vi "Config data to StepData.vi"(11 "Data":string[](array[string])) -> (3 "RootStepData":string[](array[string]))   [LabVIEW 2021, in "DataBase_SQL.lvclass"]
uses:
  <userlib>/John_Lib/DataBase/DataBase_SQL/DataBase_SQL.lvclass
  <userlib>/John_Lib/DataBase/DataBase_SQL/DataBase_SQL.lvclass/DataBase_SQL.ctl
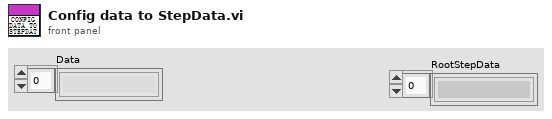
[diagram p1: front panel]
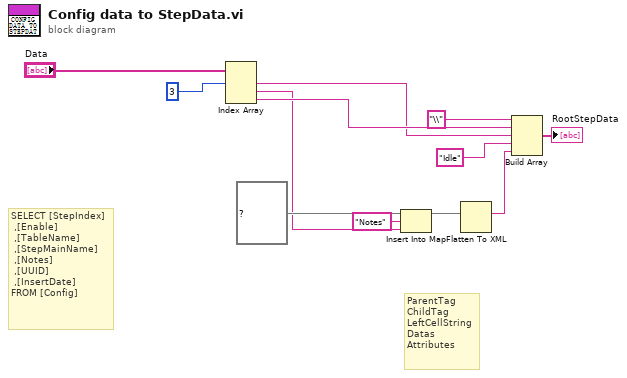
[diagram p0: block diagram]
diagram:
  # "SELECT [StepIndex]\n\t,[Enable]\n\t,[TableName]\n\t,[StepMainName]\n\t,[Notes]\n\t,[UUID]\n\t,[InsertDate]\nFROM [Config]"
  # "ParentTag\nChildTag\nLeftCellString\nDatas\nAttributes"
  n1 = Index Array(array="Data", index #1=3 ("index")) -> (element #1=w8:string, element #2=w6:string, element #3=w9:string)  [unwired: 2 in]
  n2 = Insert Into Map(map in=map{string, string} {} ("map"), key="Notes", value=w6) -> (map out=w3:map{string, string})  [unwired: 2 out]
  n3 = Flatten To XML(6:w3) -> (2:w2:string)
  n4 = Build Array("\\" ("format string"), w9, w8, "Idle" ("element"), w2) -> (→"RootStepData":string[])
